vi "Swerve Drive.vi"(5 "Rot. Point X":dbl, 6 "Auto Controls":bool, 7 "Rot. Point Y":dbl) -> ()   [LabVIEW 2019]
uses:
  Robot Global Data.vi
  <vilib>/addons/control/pid/pid.llb/PID (DBL).vi
  <vilib>/addons/control/pid/NI_PID_pid.lvlib
panel:
  out "Gyro Angle":dbl(knob)=1116.8701171875 scale=0.0..360.0
  out "Heading":dbl=1078.505859375
  in  "Maintain Z Angle PID gains":T1={"proportional gain (Kc)"=0.0045, "integral time (Ti, min)"=0.0, "derivative time (Td, min)"=0.0} {"derivative time (Td, min)" format="%.4f"; "integral time (Ti, min)" format="%.4f"; "proportional gain (Kc)" format="%.4f"}
  in  "FeedForward":dbl
  in  "fr offset":dbl(knob)=144.0 scale=-180.0..180.0
  in  "fl offset":dbl(knob)=347.0 scale=-180.0..180.0
  in  "br offset":dbl(knob)=258.0 scale=-180.0..180.0
  in  "bl offset":dbl(knob)=89.0 scale=-180.0..180.0
  in  "Robot Length":dbl=34.0
  in  "Robot Width":dbl=25.5
  # "Comp bot\nFL: -2\nFR: -2\nBL: -1\nBR: 0"
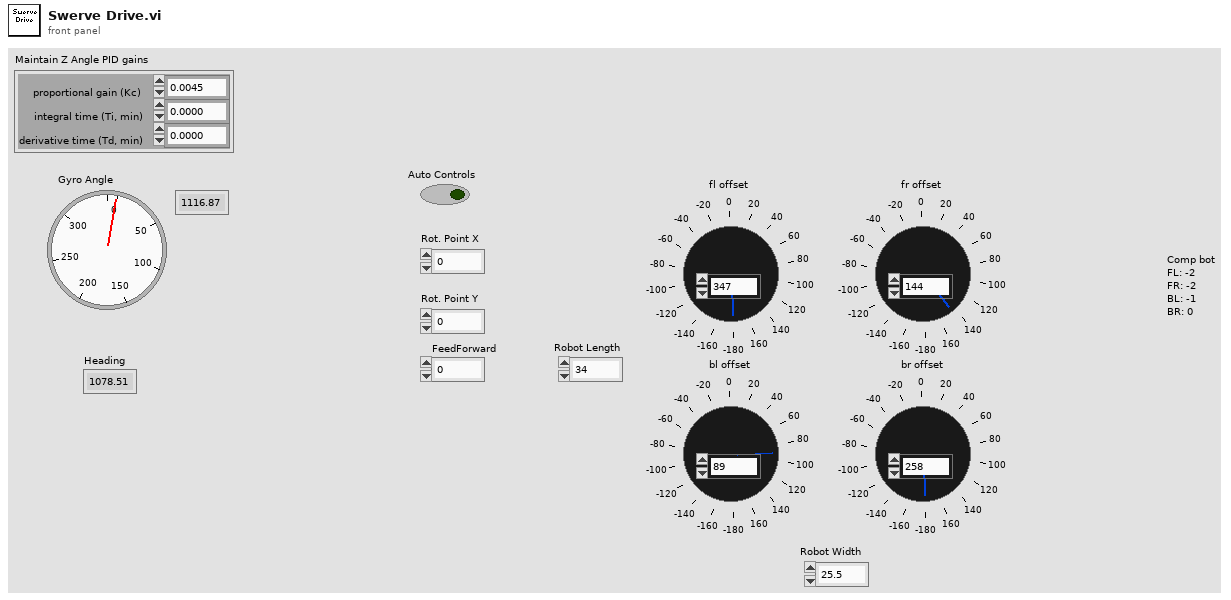
[diagram p1: front panel]
types:
  T1 = cluster{"proportional gain (Kc)":dbl, "integral time (Ti, min)":dbl, "derivative time (Td, min)":dbl}
  T2 = enum16{"Back Left", "Back Right", "Front Left", "Front Right"}
  T3 = typedef "WPI_MotorControlDeviceRef.ctl" = cluster{"DeviceStatus":errorcluster, "Type":T4, "PWM":cluster{"PWM Channel":T5, "DeadBand":T6}, "CAN":cluster{"Device Number":u8, "SetOutput VI Ref":variant, "GetOutput VI Ref":variant, "Enable VI Ref":variant, "Disable VI Ref":variant, "Data":variant}, "Invert":bool, "DIO PWM":cluster{"PWM \"Enable\" Channel":T5, "DIOChannel":T7, "PWM Rate":dbl}}
  T4 = typedef "WPI_MotorControlType.ctl" = enum16{"PWM", "CAN", "DIO PWM"}
  T5 = typedef "FPGA_DIOPWMChannel.ctl" = enum8{"PWM 0", "PWM 1", "PWM 2", "PWM 3", "PWM 4", "PWM 5", "PWM 6", "PWM 7", "PWM 8", "PWM 9", "PWM MXP 0", "PWM MXP 1", "PWM MXP 2", "PWM MXP 3", "PWM MXP 4", "PWM MXP 5", "PWM MXP 6", "PWM MXP 7", "PWM MXP 8", "PWM MXP 9", "Invalid"}
  T6 = typedef "WPI_PWMDeadband.ctl" = cluster{"Name":string, "maxPositivePwm":i32, "minPositivePwm":i32, "centerPwm":i32, "maxNegativePwm":i32, "minNegativePwm":i32, "angularRange":u16}
  T7 = typedef "FPGA_DIOChannel.ctl" = enum8{"DIO 0", "DIO 1", "DIO 2", "DIO 3", "DIO 4", "DIO 5", "DIO 6", "DIO 7", "DIO 8", "DIO 9", "DIO MXP 0", "DIO MXP 1", "DIO MXP 2", "DIO MXP 3", "DIO MXP 4", "DIO MXP 5", "DIO MXP 6", "DIO MXP 7", "DIO MXP 8", "DIO MXP 9", "DIO MXP 10", "DIO MXP 11", "DIO MXP 12", "DIO MXP 13", "DIO MXP 14", "DIO MXP 15", "SPI Port CS1", "SPI Port CS2", "SPI Port CS3", "SPI Port MISO", "SPI Port MOSI", "Invalid"}
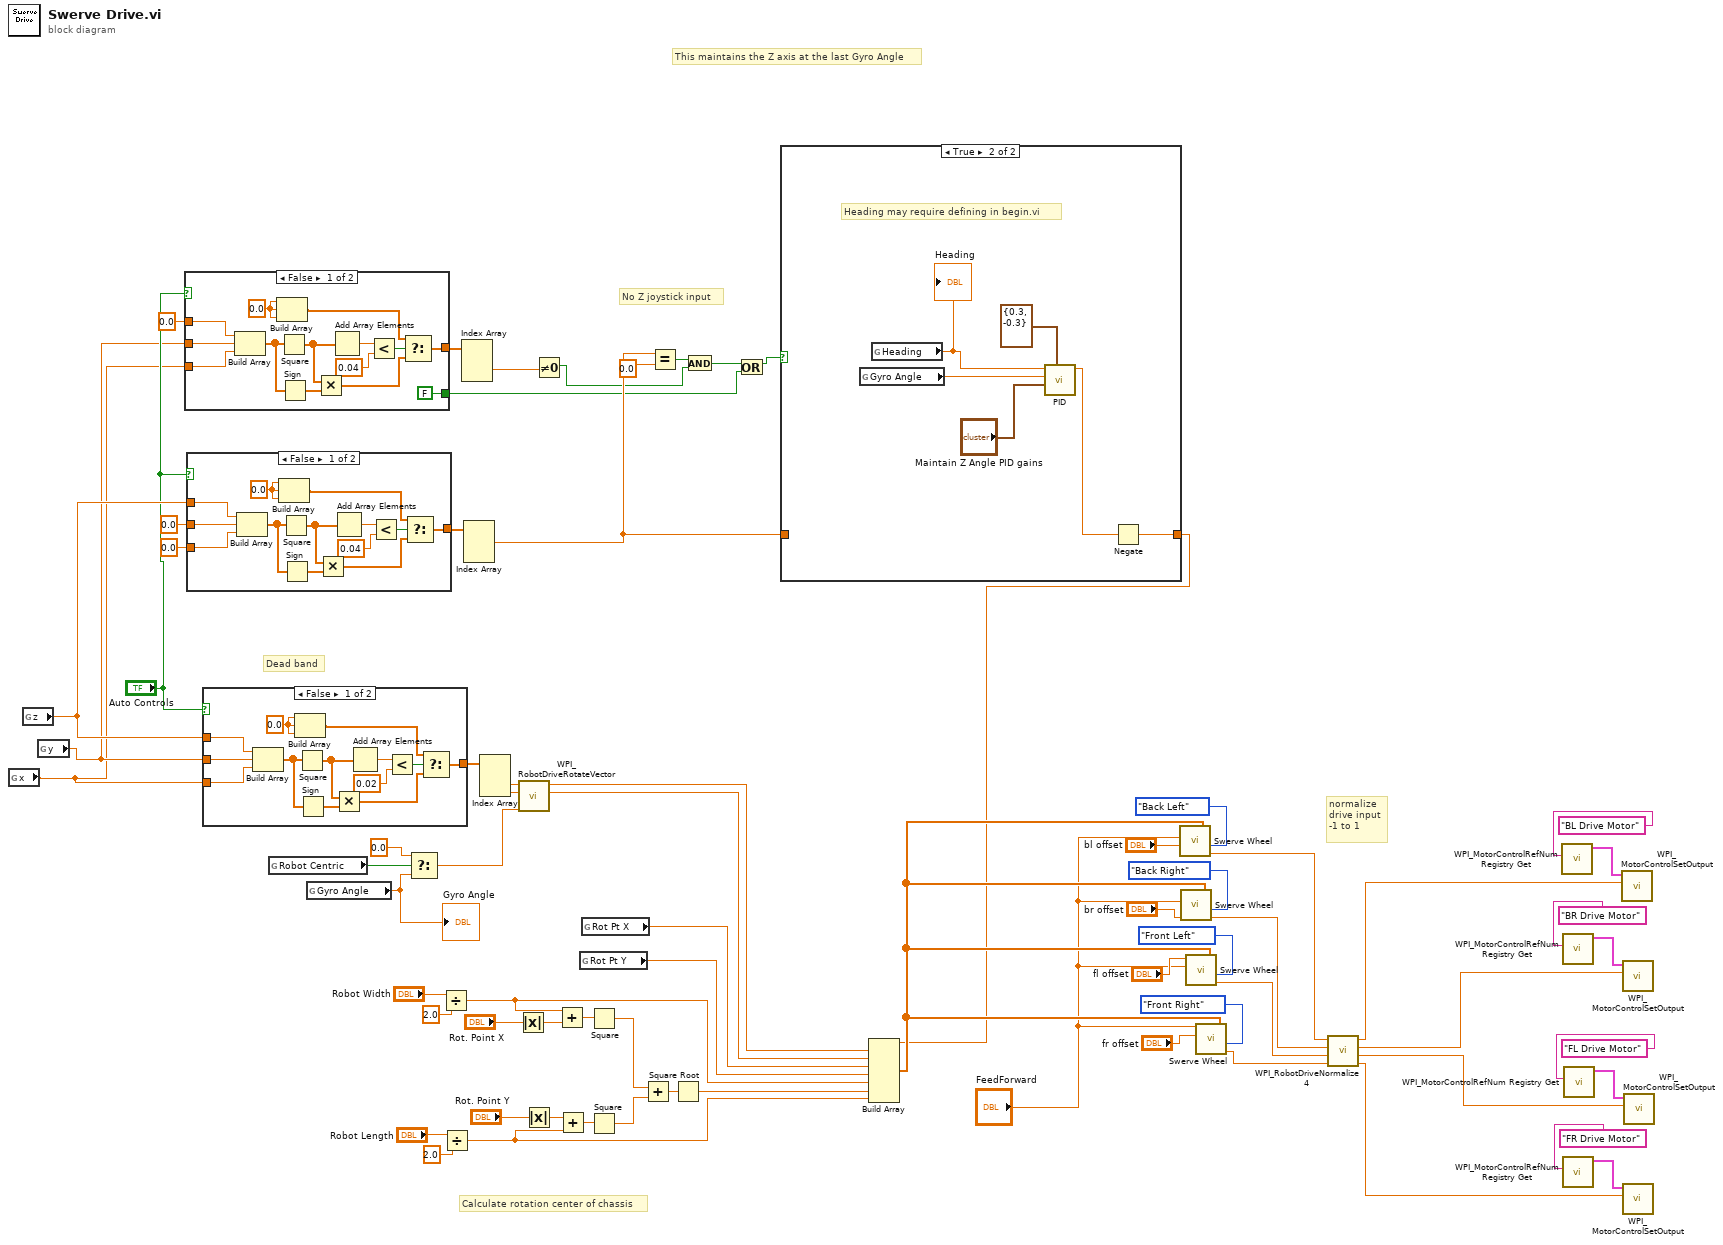
[diagram p0: block diagram]
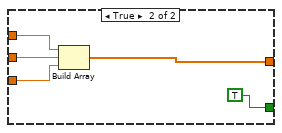
[diagram p2: hidden frame]
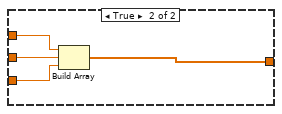
[diagram p3: hidden frame]
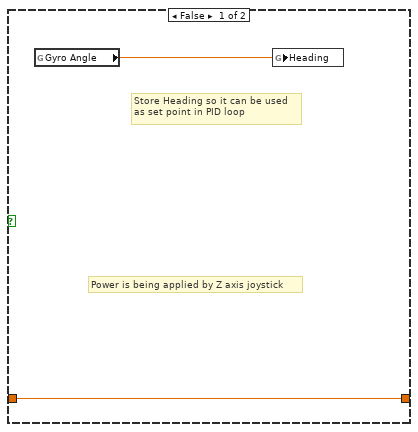
[diagram p4: hidden frame]
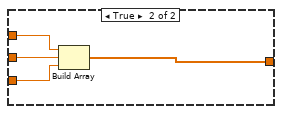
[diagram p5: hidden frame]
diagram:
  # "This maintains the Z axis at the last Gyro Angle"
  # "No Z joystick input"
  # "normalize\ndrive input\n-1 to 1"
  # "Calculate rotation center of chassis"
  # "Dead band"
  n1 = global read "Robot Global Data.vi" "x"() -> (w14:dbl)
  n2 = global read "Robot Global Data.vi" "z"() -> (w22:dbl)
  n3 = global read "Robot Global Data.vi" "y"() -> (w15:dbl)
  n4 = case shown="False" "Auto Controls" {
    tunnel: w15 -> [w73 w89]
    tunnel: w14 -> [w77 w90]
    tunnel: 0.0 ("z") -> [w74 w87]
    tunnel: [w75 w88] -> w18
    tunnel: [FALSE TRUE] -> w9
    frame False {
      w81 = 0.0 ("element")
      n5 = Build Array(w74, w73, w77) -> (w80:dbl[])
      n6 = Build Array(w81, w81, w81) -> (w82:dbl[])
      n7 = Square(x=w80) -> (x^2=w78:dbl[])
      n8 = Sign(1:w80) -> (0:w79:dbl[])
      n9 = Multiply(x=w78, y=w79) -> (x*y=w76:dbl[])
      n10 = Add Array Elements(numeric array=w78) -> (sum=w85:dbl)
      n11 = Less?(x=w85, y=0.04 ("x")) -> (x < y?=w83:bool)
      n12 = Select(t=w82, s=w83, f=w76) -> (s? t:f=w75:dbl[])
    }
    frame True {
      n13 = Build Array(w87, w89, w90) -> (w88:dbl[])
    }
  }
  n14 = case shown="False" "Auto Controls" {
    tunnel: 0.0 ("y") -> [w91 w106]
    tunnel: 0.0 ("x") -> [w95 w107]
    tunnel: w22 -> [w92 w104]
    tunnel: [w93 w105] -> w21
    frame False {
      w99 = 0.0 ("element")
      n15 = Build Array(w92, w91, w95) -> (w98:dbl[])
      n16 = Build Array(w99, w99, w99) -> (w100:dbl[])
      n17 = Square(x=w98) -> (x^2=w96:dbl[])
      n18 = Sign(1:w98) -> (0:w97:dbl[])
      n19 = Multiply(x=w96, y=w97) -> (x*y=w94:dbl[])
      n20 = Add Array Elements(numeric array=w96) -> (sum=w103:dbl)
      n21 = Less?(x=w103, y=0.04 ("x")) -> (x < y?=w101:bool)
      n22 = Select(t=w100, s=w101, f=w94) -> (s? t:f=w93:dbl[])
    }
    frame True {
      n23 = Build Array(w104, w106, w107) -> (w105:dbl[])
    }
  }
  n24 = case shown="False" "Auto Controls" {
    tunnel: w15 -> [w109 w123]
    tunnel: w14 -> [w113 w124]
    tunnel: w22 -> [w110 w121]
    tunnel: [w111 w122] -> w67
    frame False {
      w117 = 0.0 ("element")
      n25 = Build Array(w110, w109, w113) -> (w116:dbl[])
      n26 = Build Array(w117, w117, w117) -> (w118:dbl[])
      n27 = Square(x=w116) -> (x^2=w114:dbl[])
      n28 = Sign(1:w116) -> (0:w115:dbl[])
      n29 = Multiply(x=w114, y=w115) -> (x*y=w112:dbl[])
      n30 = Add Array Elements(numeric array=w114) -> (sum=w120:dbl)
      n31 = Less?(x=w120, y=0.02 ("x")) -> (x < y?=w108:bool)
      n32 = Select(t=w118, s=w108, f=w112) -> (s? t:f=w111:dbl[])
    }
    frame True {
      n33 = Build Array(w121, w123, w124) -> (w122:dbl[])
    }
  }
  n34 = global read "Robot Global Data.vi" "Robot Centric"() -> (w66:bool)
  n35 = global read "Robot Global Data.vi" "Gyro Angle"() -> (w64:dbl)
  "Gyro Angle" <- w64
  n36 = Select(t=0.0, s=w66, f=w64) -> (s? t:f=w61:dbl)
  n37 = Divide(x="Robot Width", y=2.0) -> (x/y=w46:dbl)
  n38 = Divide(x="Robot Length", y=2.0) -> (x/y=w48:dbl)
  n39 = Index Array(array=w18) -> (element #2=w13:dbl)  [unwired: 3 in, 2 out]
  n40 = Index Array(array=w21) -> (element #1=w20:dbl)  [unwired: 3 in, 2 out]
  n41 = Index Array(array=w67) -> (element #2=w63:dbl, element #3=w62:dbl)  [unwired: 3 in, 1 out]
  n42 = Absolute Value(x="Rot. Point X") -> (abs(x)=w60:dbl)
  n43 = call "WPI_RobotDriveRotateVector.vi"("Angle"=w61, "X"=w62, "Y"=w63) -> ("X'"=w43:dbl, "Y'"=w42:dbl)  [unwired: 7 in]
  n44 = Absolute Value(x="Rot. Point Y") -> (abs(x)=w58:dbl)
  n45 = Not Equal To 0?(x=w13) -> (x != 0?=w12:bool)
  n46 = Add(x=w46, y=w60) -> (x+y=w59:dbl)
  n47 = Add(x=w58, y=w48) -> (x+y=w57:dbl)
  n48 = global read "Robot Global Data.vi" "Rot Pt Y"() -> (w45:dbl)
  n49 = global read "Robot Global Data.vi" "Rot Pt X"() -> (w44:dbl)
  n50 = Square(x=w59) -> (x^2=w55:dbl)
  n51 = Square(x=w57) -> (x^2=w56:dbl)
  n52 = Add(x=w55, y=w56) -> (x+y=w54:dbl)
  n53 = Equal?(x=w20, y=0.0) -> (x = y?=w19:bool)
  n54 = Square Root(x=w54) -> (sqrt(x)=w47:dbl)
  n55 = And(x=w19, y=w12) -> (x .and. y?=w11:bool)
  n56 = Or(x=w11, y=w9) -> (x .or. y?=w10:bool)
  n57 = case shown="True" w10 {
    tunnel: w20 -> [w125 _]
    tunnel: [w125 w127] -> w25
    frame False {
      # "Store Heading so it can be used\nas set point in PID loop"
      # "Power is being applied by Z axis joystick"
      n58 = global read "Robot Global Data.vi" "Gyro Angle"() -> (w126:dbl)
      n59 = global write "Robot Global Data.vi" "Heading"(w126) -> ()
    }
    frame True {
      # "Heading may require defining in begin.vi"
      n60 = global read "Robot Global Data.vi" "Gyro Angle"() -> (w131:dbl)
      n61 = global read "Robot Global Data.vi" "Heading"() -> (w130:dbl)
      "Heading" <- w130
      n62 = call-poly <vilib>:"PID.vi"("output range"=cluster{"output high":dbl, "output low":dbl} {"output high"=0.3, "output low"=-0.3}, "PID gains"="Maintain Z Angle PID gains", "process variable"=w131, "setpoint"=w130) -> ("output"=w128:dbl)  [unwired: 6 in, 1 out]
      n63 = Negate(x=w128) -> (-x=w127:dbl)
    }
  }
  n64 = Build Array(w25, w42, w43, w44, w45, w46, w47, w48) -> (w31:dbl[])
  n65 = call "Swerve Wheel.vi"("Wheel"=T2."Back Left", "FeedForward"="FeedForward", "Inputs"=w31, "bl offset"="bl offset") -> ("Speed"=w39:dbl)  [unwired: 3 in]
  n66 = call "Swerve Wheel.vi"("Wheel"=T2."Back Right", "FeedForward"="FeedForward", "Inputs"=w31, "br offset"="br offset") -> ("Speed"=w34:dbl)  [unwired: 3 in]
  n67 = call "Swerve Wheel.vi"("Wheel"=T2."Front Left", "FeedForward"="FeedForward", "Inputs"=w31, "fl offset"="fl offset") -> ("Speed"=w33:dbl)  [unwired: 3 in]
  n68 = call "Swerve Wheel.vi"("Wheel"=T2."Front Right", "FeedForward"="FeedForward", "Inputs"=w31, "fr offset"="fr offset") -> ("Speed"=w32:dbl)  [unwired: 3 in]
  n69 = call "WPI_RobotDriveNormalize 4.vi"("D"=w32, "C"=w33, "B"=w34, "A"=w39) -> ("D'"=w68:dbl, "C'"=w69:dbl, "B'"=w70:dbl, "A'"=w71:dbl)
  n70 = call <vilib>:"WPI_MotorControlRefNum Registry Get.vi"("refnum name"="BL Drive Motor") -> ("MotorControlDevRef"=w8:T3)  [unwired: 9 in, 1 out]
  n71 = call <vilib>:"WPI_MotorControlRefNum Registry Get.vi"("refnum name"="BR Drive Motor") -> ("MotorControlDevRef"=w7:T3)  [unwired: 9 in, 1 out]
  n72 = call <vilib>:"WPI_MotorControlRefNum Registry Get.vi"("refnum name"="FR Drive Motor") -> ("MotorControlDevRef"=w5:T3)  [unwired: 9 in, 1 out]
  n73 = call <vilib>:"WPI_MotorControlRefNum Registry Get.vi"("refnum name"="FL Drive Motor") -> ("MotorControlDevRef"=w6:T3)  [unwired: 9 in, 1 out]
  n74 = call <vilib>:"WPI_MotorControlSetOutput.vi"("Output"=w71, "MotorControlDevRef"=w8) -> ()  [unwired: 7 in, 3 out]
  n75 = call <vilib>:"WPI_MotorControlSetOutput.vi"("Output"=w70, "MotorControlDevRef"=w7) -> ()  [unwired: 7 in, 3 out]
  n76 = call <vilib>:"WPI_MotorControlSetOutput.vi"("Output"=w68, "MotorControlDevRef"=w5) -> ()  [unwired: 7 in, 3 out]
  n77 = call <vilib>:"WPI_MotorControlSetOutput.vi"("Output"=w69, "MotorControlDevRef"=w6) -> ()  [unwired: 7 in, 3 out]
